vi "PicoScope6000aSetDataBuffers.vi"(5 "enabled array":i16[](array[numeric]), 7 "Buffer and Transfer Settings":T2 {"Down-Sample Mode" items=["None", "Aggregate", "Decimate", "Average"]; "Down Sample Ratio" step=1; "Samples" format="%_6p"}, 8 "error in (no error)":errorcluster, 10 "Data Pointers In":T1, 11 "handle in":i16) -> (0 "error out":errorcluster, 3 "handle out":i16)   [LabVIEW 2009]
doc: "Calls ps6000aSetDataBuffers, and assigns Pico buffers"
uses:
  ps6000a.dll
  shared/PicoBuffers.ctl
panel:
  out "Actionflag":bool
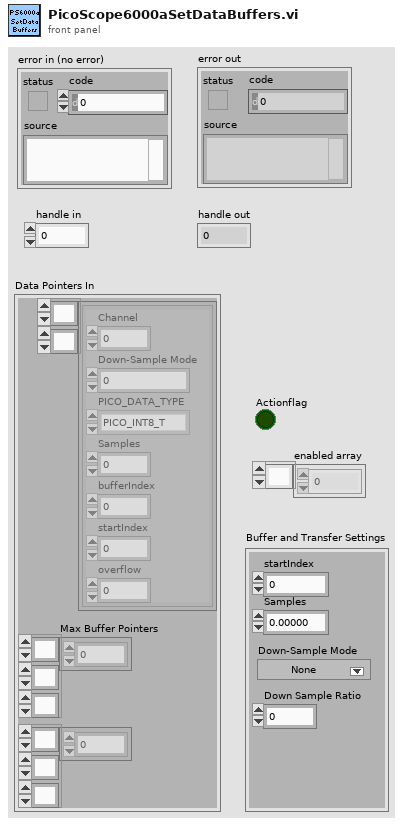
[diagram p1: front panel]
types:
  T1 = typedef "PicoBuffers.ctl" = cluster{"Max Buffer Pointers":u64[][][], "Min Buffer Pointers":u64[][][], "StreamingDataInfo":cluster{"Channel":u32, "Down-Sample Mode":u32, "PICO_DATA_TYPE":enum32{"PICO_INT8_T", "PICO_INT16_T", "PICO_INT32_T", "PICO_UINT32_T", "PICO_INT64_T", ""}, "Samples":i32, "bufferIndex":u64, "startIndex":i32, "overflow":i16}[][]}
  T2 = cluster{"startIndex":u64, "Samples":u64, "Down Sample Ratio":u64, "Down-Sample Mode":u32}
  T3 = enum32{"PICO_INT8_T", "PICO_INT16_T", "PICO_INT32_T", "PICO_UINT32_T", "PICO_INT64_T", ""}
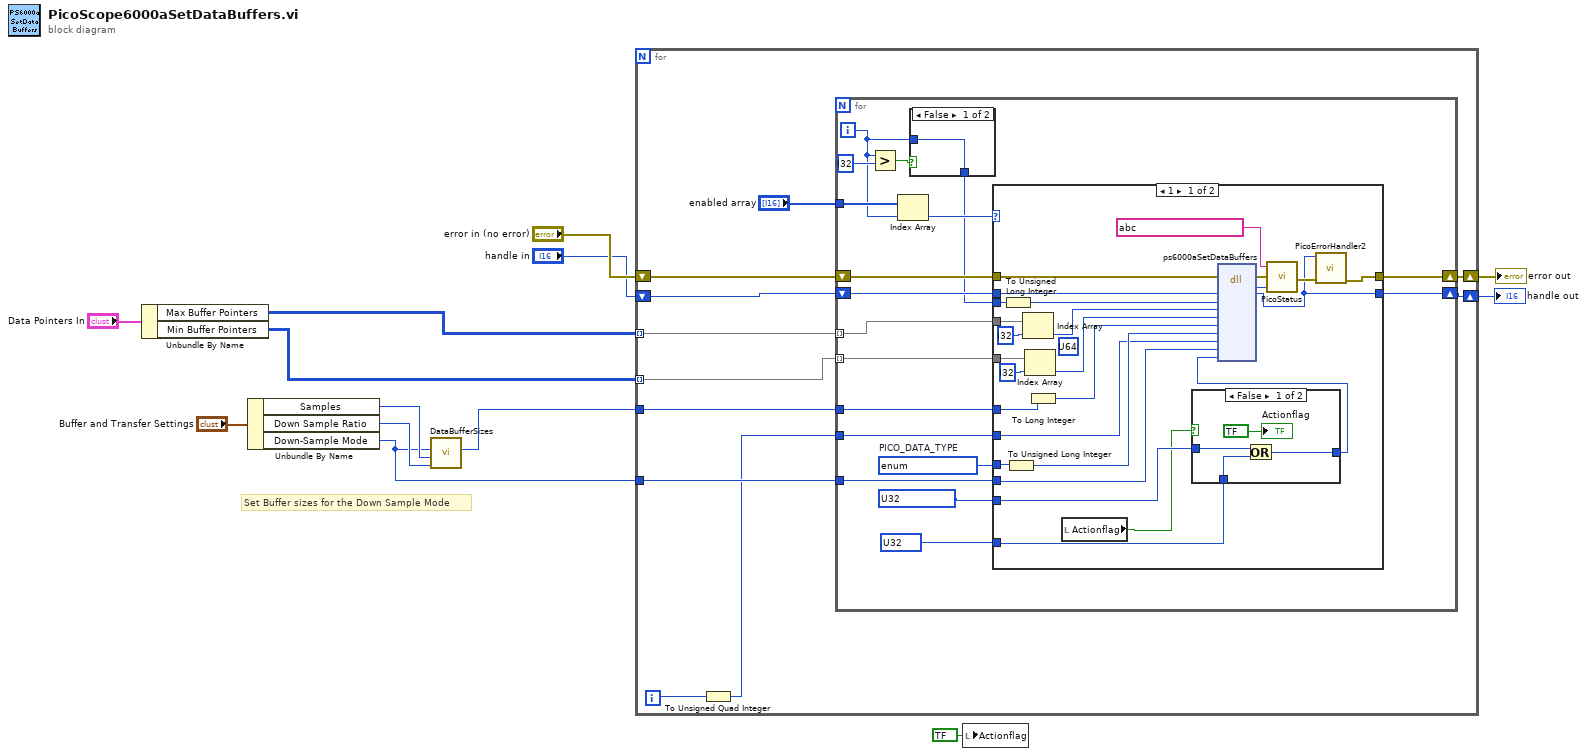
[diagram p0: block diagram]
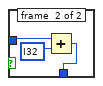
[diagram p4: hidden frame]
diagram:
  # "Set Buffer sizes for the Down Sample Mode"
  n1 = Unbundle By Name("Data Pointers In") -> ("Max Buffer Pointers"=w2:u64[][][], "Min Buffer Pointers"=w1:u64[][][])
  n2 = Unbundle By Name("Buffer and Transfer Settings") -> ("Samples"=w5:u64, "Down Sample Ratio"=w6:u64, "Down-Sample Mode"=w4:u32)
  n3 = call "DataBufferSizes.vi"("Down Sample Ratio"=w6, "Number of Samples"=w5, "Down-Sample Mode"=w4) -> ("Max Buffer Size"=w7:i32)  [unwired: 7 in, 1 out]
  n4 = for {
    tunnel: w7 -> [w20]
    tunnel: w4 -> [w19]
    tunnel: w2 -> [w18] mode=indexing
    tunnel: w1 -> [w17] mode=indexing
    shift-right: [w24] -> w12
    shift-left: "error in (no error)" -> [w22]
    shift-right: [w23] -> w11
    shift-left: "handle in" -> [w21]
    i -> [w14]
    n5 = To Unsigned Quad Integer(1:w14) -> (0:w15:u64)
    n6 = for {
      tunnel: w19 -> [w42]
      tunnel: w20 -> [w34]
      tunnel: "enabled array" -> [w39]
      tunnel: w18 -> [w33] mode=indexing
      shift-right: [w32] -> w24
      shift-left: w22 -> [w41]
      tunnel: w17 -> [w27] mode=indexing
      shift-right: [w26] -> w23
      shift-left: w21 -> [w40]
      tunnel: w15 -> [w25]
      i -> [w31]
      w28 = T3 ?  # PICO_DATA_TYPE
      w29 = u32 ? items=["NONE", "CLEAR_ALL", "ADD", "CLEAR_THIS_DATA_BUFFER", "CLEAR_WAVEFORM_DATA_BUFFERS", "CLEAR_WAVEFORM_READ_DATA_BUFFERS"] ("PicoAction 1")
      w30 = u32 ? items=["NONE", "CLEAR_ALL", "ADD", "CLEAR_THIS_DATA_BUFFER", "CLEAR_WAVEFORM_DATA_BUFFERS", "CLEAR_WAVEFORM_READ_DATA_BUFFERS"] ("PicoAction 2")
      n7 = Greater?(x=w31, y=i32 ?) -> (0:w36:bool)
      n8 = Index Array(array=w39, index=w31) -> (element=w38:i16)
      n9 = case shown="False" w36 {
        tunnel: [w76 w77] -> w35
        tunnel: w31 -> [w76 w79]
        frame #0 {
        }
        frame #1 {
          n10 = Add(x=w79, y=i32 ?) -> (x+y=w77:i32)
        }
      }
      n11 = case shown="1" w38 {
        tunnel: w35 -> [w57 _]
        tunnel: w41 -> [w68 w75]
        tunnel: w40 -> [w65 w74]
        tunnel: w42 -> [w62 _]
        tunnel: w28 -> [w48 _]
        tunnel: w29 -> [w52 _]
        tunnel: [w61 w75] -> w32
        tunnel: [w60 w74] -> w26
        tunnel: w34 -> [w59 _]
        tunnel: w33 -> [w53 _]
        tunnel: w30 -> [w51 _]
        tunnel: w27 -> [w45 _]
        tunnel: w25 -> [w43 _]
        frame #0 {
          (unwired) u64 ? ("waveform")
          n12 = To Unsigned Long Integer(number=w57) -> (unsigned 32bit integer=w56:u32)
          n13 = To Unsigned Long Integer(number=w48) -> (unsigned 32bit integer=w49:u32)
          n14 = Index Array(array=w53, index=i32 ?) -> (element=w54:u64)
          n15 = Index Array(array=w45, index=i32 ?) -> (element=w46:u64)
          n16 = To Long Integer(number=w59) -> (32bit integer=w58:i32)
          n17 = local read "Actionflag"() -> (w44:bool)
          n18 = case shown="False" w44 {
            tunnel: w52 -> [w72 _]
            tunnel: w51 -> [w71 w73]
            tunnel: [w70 w73] -> w50
            frame #0 {
              n19 = Or(x=w72, y=w71) -> (x .or. y?=w70:u32)
              "Actionflag" <- bool ? ("Actionflag")
            }
            frame #1 {
            }
          }
          n20 = dll-call lib="ps6000a.dll" fn="ps6000aSetDataBuffers" ("ps3000.dll:_ps3000_open_unit@0")(error in=w68, "handle"=w65, "channel"=w56, "bufferMax"=w54, "bufferMin"=w46, "nSamples"=w58, "dataType"=w49, "waveform"=w43, "downSampleRatioMode"=w62, "action"=w50) -> (error out=w67:errorcluster, "PICO_STATUS"=w66:u32, "handle"=w60:i16)  [unwired: 10 in, 1 out]
          n21 = call "PicoStatus.vi"("PICO STATUS"=w66, "error in"=w67, "source"=string ?) -> ("error out"=w63:errorcluster)
          n22 = call "PicoErrorHandler2.vi"("error in (no error)"=w63, "handle In"=w60) -> ("error out"=w61:errorcluster)  [unwired: 9 in]
        }
        frame #1 {
        }
      }
    }
  }
  "error out" <- w12
  "handle out" <- w11
  n23 = local write "Actionflag"(bool ? ("Actionflag")) -> ()
